vi "Drawer.vi"() -> ()   [LabVIEW 2014]
uses:
  <vilib>/Utility/file.llb/Read From Spreadsheet File (I64).vi
  <vilib>/Utility/file.llb/Read From Spreadsheet File (DBL).vi
panel:
  out "size(s)":i32
  out "HF/LF_ERP":dbl[][](graph)
  out "PPI_ERP":dbl[][](graph)
  out "HF_ERP":dbl[][](graph)
  out "LF_ERP":dbl[][](graph)
  out "VLF_ERP":dbl[][](graph)
  in  "Trial_number":i32
  in  "stop":bool
  in  "피험자_이름":string
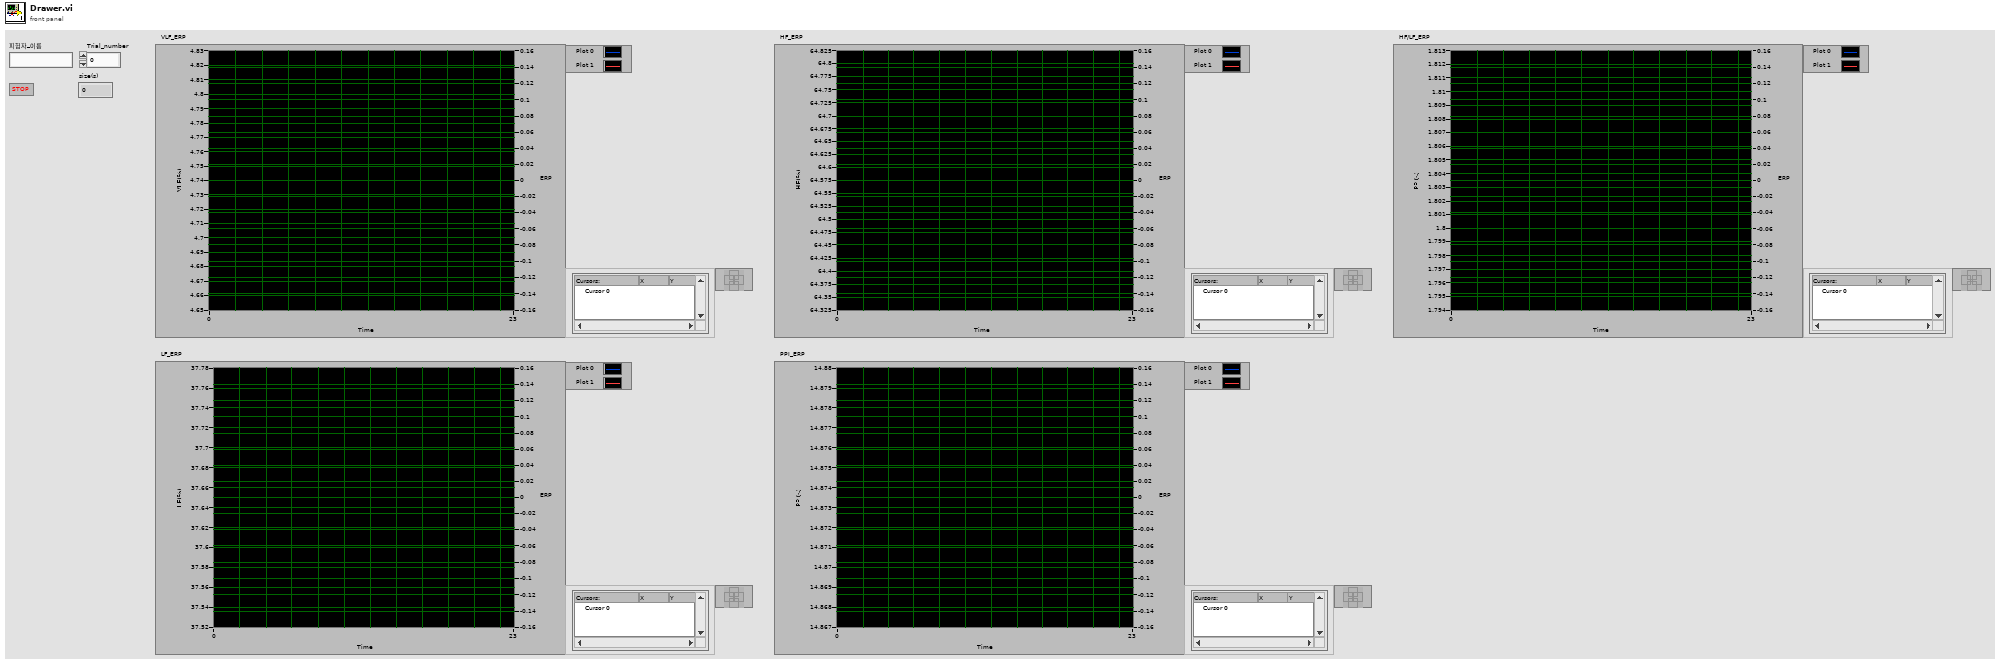
[diagram p1: front panel]
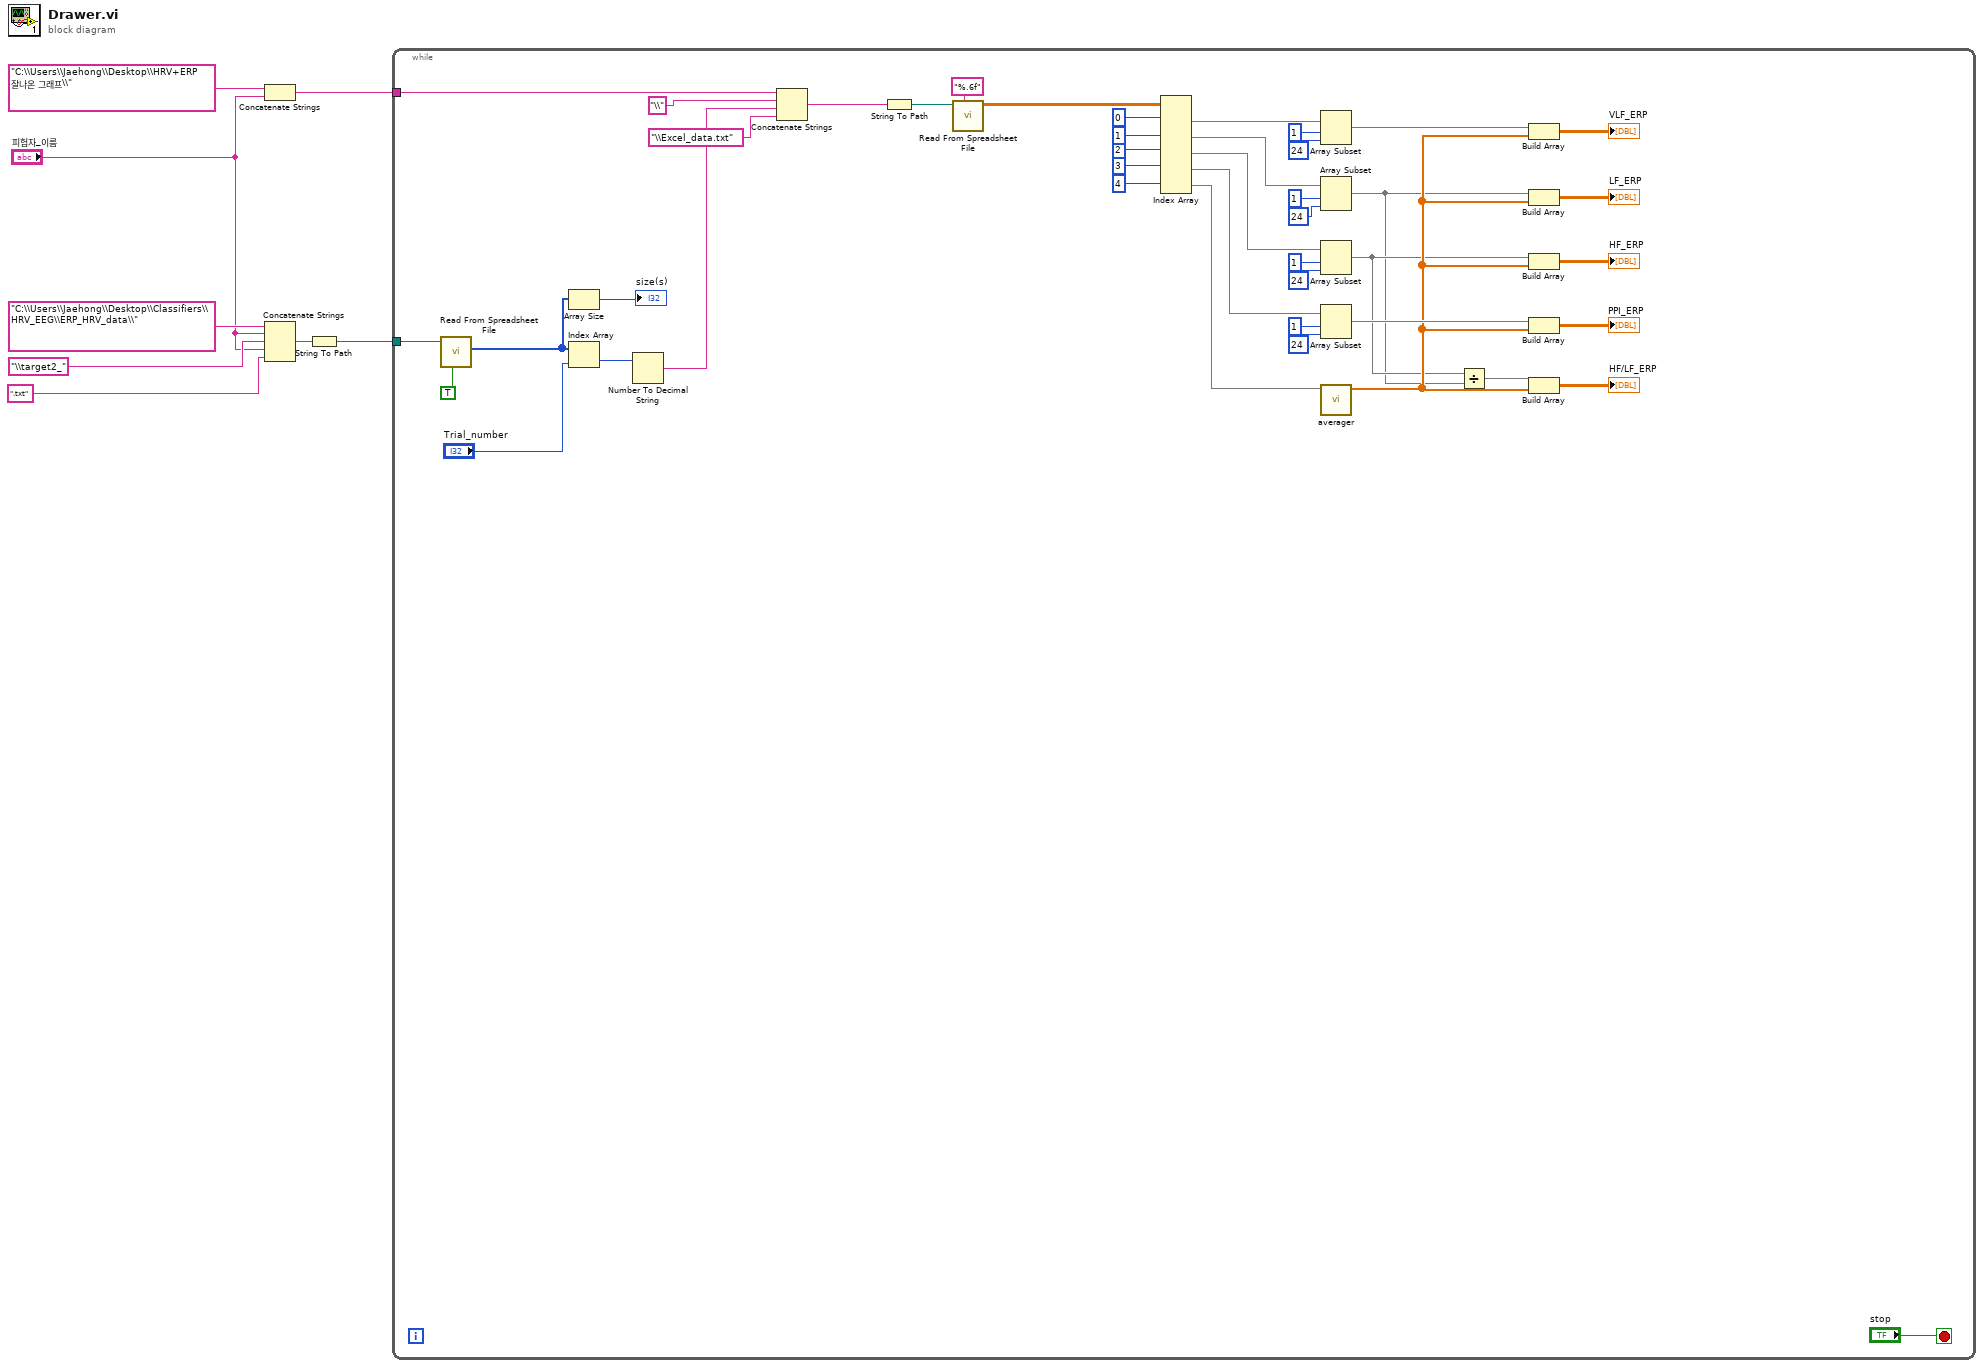
[diagram p0: block diagram]
diagram:
  n1 = Concatenate Strings("C:\\Users\\Jaehong\\Desktop\\HRV+ERP 잘나온 그래프\\", "피험자_이름") -> (w7:string)
  n2 = Concatenate Strings("C:\\Users\\Jaehong\\Desktop\\Classifiers\\HRV_EEG\\ERP_HRV_data\\", "피험자_이름", "\\target2_", "피험자_이름", ".txt") -> (w2:string)
  n3 = String To Path(string=w2) -> (path=w1:path)
  n4 = while {
    tunnel: w7 -> [w48]
    tunnel: w1 -> [w52]
    stop <- "stop" stop-if-true
    n5 = call-poly <vilib>:"Read From Spreadsheet File.vi"("transpose (no:F)"=TRUE, "file path (dialog if empty)"=w52) -> ("first row"=w10:i64[])  [unwired: 5 in, 4 out]
    n6 = Array Size(array=w10) -> (size(s)=→"size(s)":i32)
    n7 = Index Array(array=w10, index="Trial_number") -> (element=w46:i64)
    n8 = Number To Decimal String(number=w46) -> (decimal integer string=w45:string)  [unwired: 1 in]
    n9 = Concatenate Strings(w48, "\\", w45, "\\Excel_data.txt") -> (w43:string)
    n10 = String To Path(string=w43) -> (path=w42:path)
    n11 = call-poly <vilib>:"Read From Spreadsheet File.vi"("format (%.3f)"="%.6f", "file path (dialog if empty)"=w42) -> ("all rows"=w40:dbl[][])  [unwired: 5 in, 4 out]
    n12 = Index Array(array=w40, index (row) #1=0 ("index (row)"), index (row) #2=1 ("index (row)"), index (row) #3=2 ("index (row)"), index (row) #4=3 ("index (row)"), index (row) #5=4 ("index (row)")) -> (element #1=w34:dbl[], element #2=w25:dbl[], element #3=w24:dbl[], element #4=w23:dbl[], element #5=w22:dbl[])  [unwired: 5 in]
    n13 = Array Subset(array=w34, index=1, length=24) -> (w21:dbl[])
    n14 = Array Subset(array=w25, index=1, length=24) -> (w11:dbl[])
    n15 = Array Subset(array=w24, index=1, length=24) -> (w12:dbl[])
    n16 = Array Subset(array=w23, index=1, length=24) -> (w20:dbl[])
    n17 = call "averager.vi"("input"=w22) -> ("output"=w14:dbl[])  [unwired: 10 in]
    n18 = Divide(x=w12, y=w11) -> (x/y=w13:dbl[])
    n19 = Build Array(w21, w14) -> (→"VLF_ERP":dbl[][])
    n20 = Build Array(w11, w14) -> (→"LF_ERP":dbl[][])
    n21 = Build Array(w12, w14) -> (→"HF_ERP":dbl[][])
    n22 = Build Array(w20, w14) -> (→"PPI_ERP":dbl[][])
    n23 = Build Array(w13, w14) -> (→"HF/LF_ERP":dbl[][])
  }
